vi "Main.vi"() -> ()   [LabVIEW 2013]
doc: "该连续测量范例项目在队列消息处理器模板的基础上实现。\n\n事件处理循环负责按用户界面操作生成对应的消息。\n\n消息处理循环负责对事件处理循环或其他消息生成的消息进行处理。其中还包括用于采集和记录消息处理循环的子VI，以及用于更新图表的循环。"
uses:
  Settings/Settings.ctl
  Acquisition/Hardware Configuration.ctl
  Acquisition/Signal Type.ctl
  Logging/Logging Configuration.ctl
  controls/UI Data.ctl
  controls/UI State.ctl
  support/Message Queue/Enqueue Message (Single).vi
  support/Message Queue/Enqueue Message (Array).vi
  <vilib>/Utility/error.llb/Error Cluster From Error Code.vi
  <vilib>/ErrorRing/Error Ring.xnode
  Acquisition/Acquisition.lvlib
  Logging/Logging.lvlib
  Settings/Settings.lvlib
  support/User Event - Stop/User Event - Stop.lvlib
  support/Message Queue/Message Queue.lvlib
panel:
  out "数据":waveform(dbl)[](graph)
  in  "设置":bool
  in  "开始":bool
  in  "停止":bool
  out "状态":string
  in  "退出":bool
  # "连续测量数据记录器"
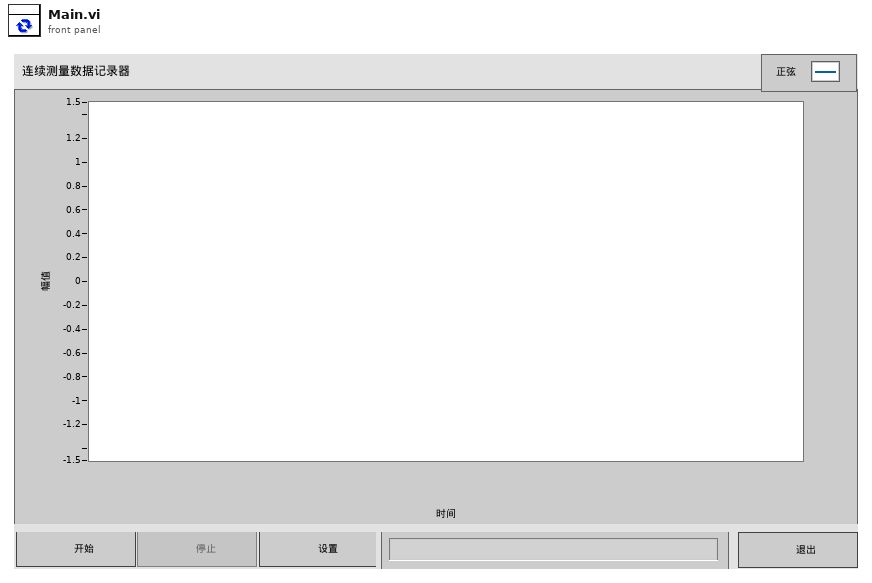
[diagram p1: front panel]
types:
  T1 = typedef "UI State.ctl" = enum16{"Idle", "Acquiring and Logging", "Waiting for Exit", "Waiting for Exit (Acq Stopped)", "Waiting for Exit (Log Stopped)", "Waiting for Stop", "Waiting for Stop (Acq Stopped)", "Waiting for Stop (Log Stopped)"}
  T2 = typedef "UI Data.ctl" = cluster{"开始引用":refnum<vi>, "停止引用":refnum<vi>, "设置引用":refnum<vi>, "退出引用":refnum<vi>, "状态引用":refnum<vi>, "数据引用":refnum<vi>}
  T3 = typedef "Settings.lvlib/Settings.ctl" = cluster{"硬件配置":T4, "记录配置":T6}
  T4 = typedef "Acquisition.lvlib/Hardware Configuration.ctl" = cluster{"硬件引用句柄<替换此项>":string, "信号类型<替换该项>":T5}
  T5 = typedef "Acquisition.lvlib/Signal Type.ctl" = enum16{"Sine Wave", "Square with Noise"}
  T6 = typedef "Logging.lvlib/Logging Configuration.ctl" = cluster{"记录文件基路径":path, "TDMS文件引用":refnum<k34>}
  T7 = typedef "Message Queue.lvlib/All Message Queues.ctl" = cluster{"UI":refnum<queue>, "采集":refnum<queue>, "记录":refnum<queue>}
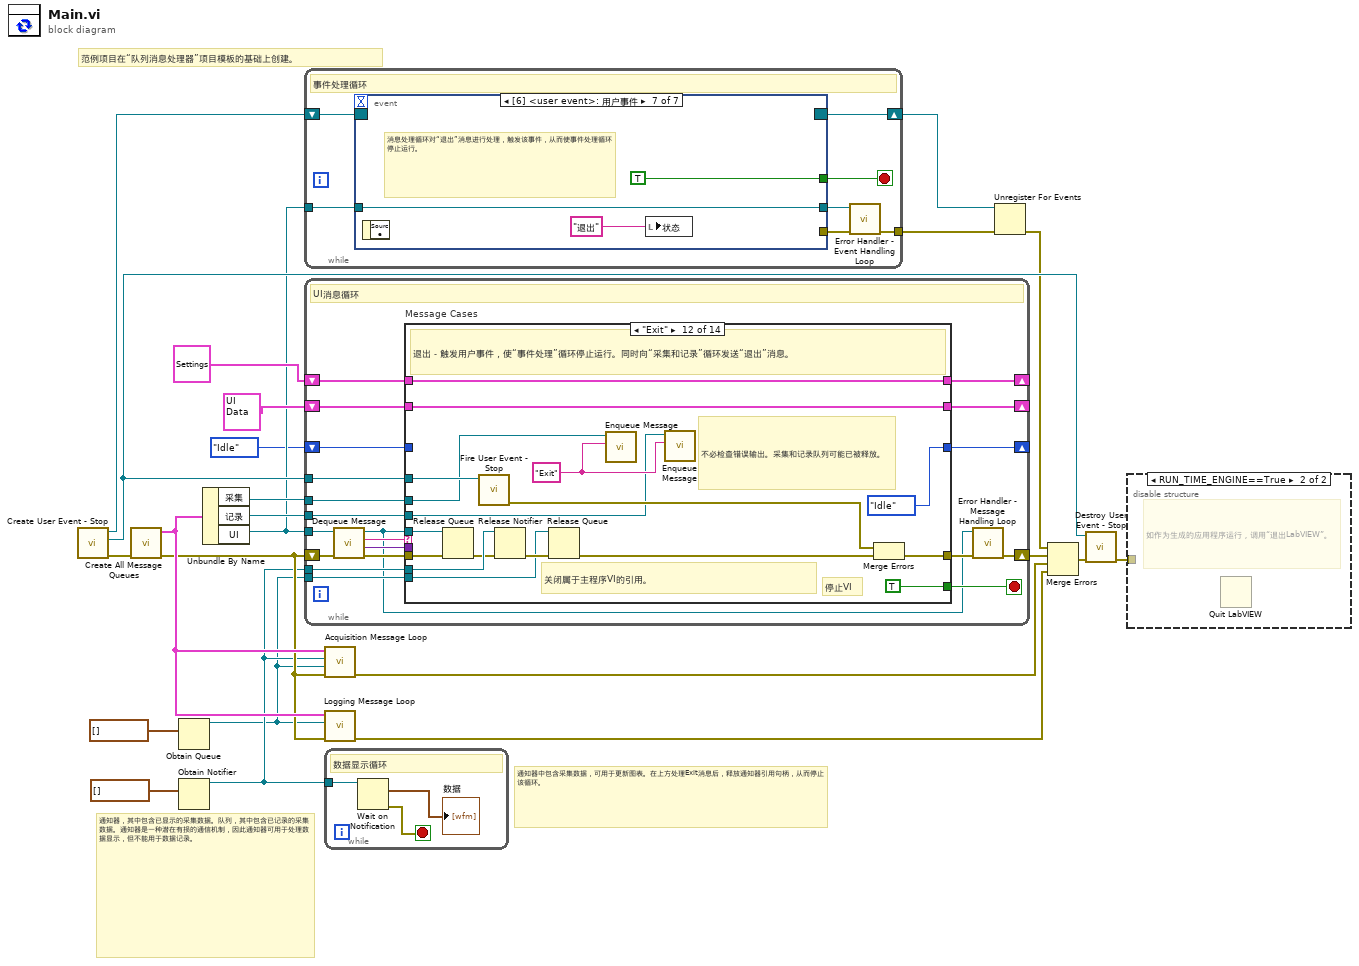
[diagram p0: block diagram]
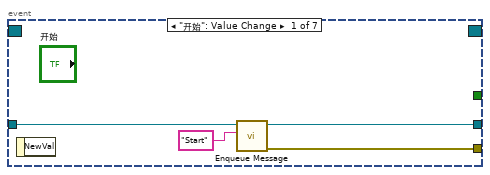
[diagram p3: hidden frame]
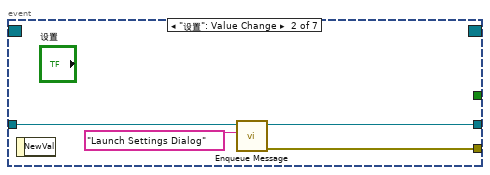
[diagram p4: hidden frame]
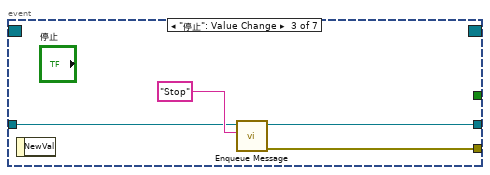
[diagram p5: hidden frame]
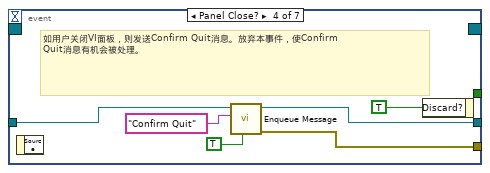
[diagram p6: hidden frame]
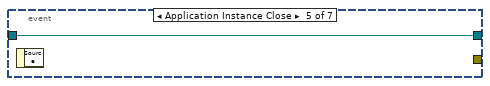
[diagram p7: hidden frame]
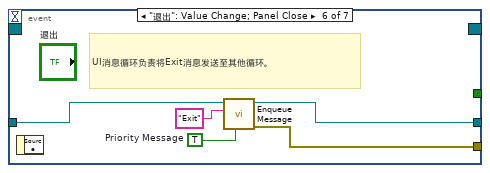
[diagram p8: hidden frame]
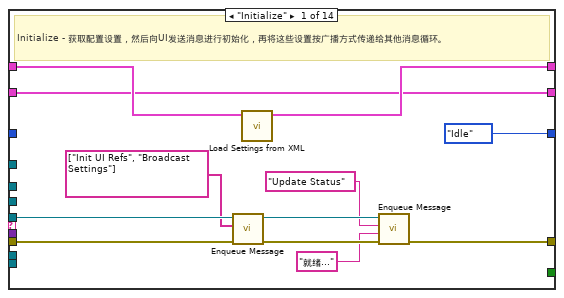
[diagram p9: hidden frame]
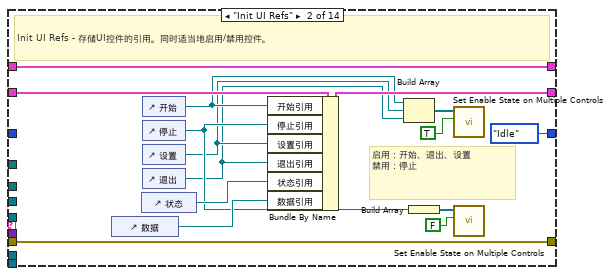
[diagram p10: hidden frame]
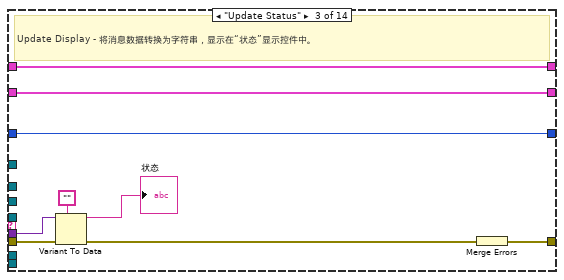
[diagram p11: hidden frame]
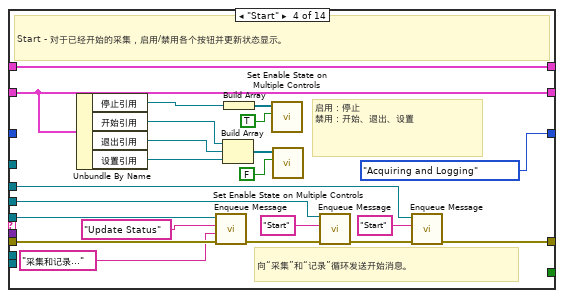
[diagram p12: hidden frame]
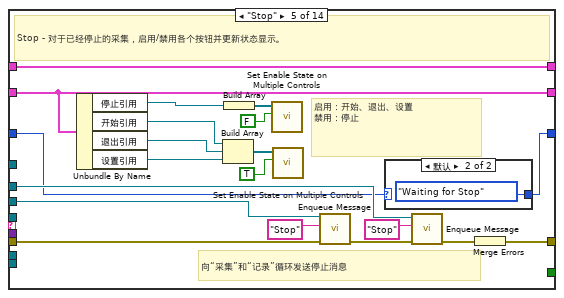
[diagram p13: hidden frame]
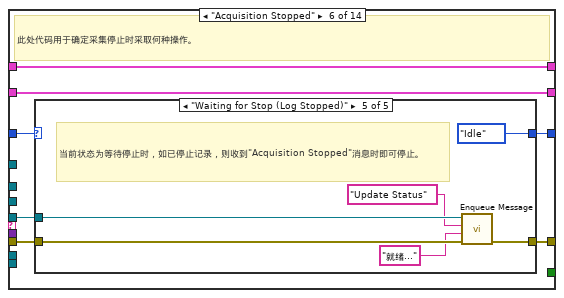
[diagram p15: hidden frame]
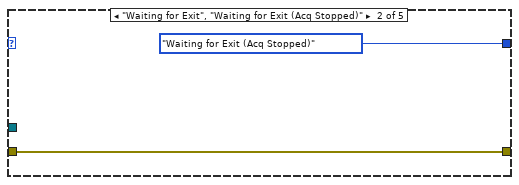
[diagram p17: hidden frame]
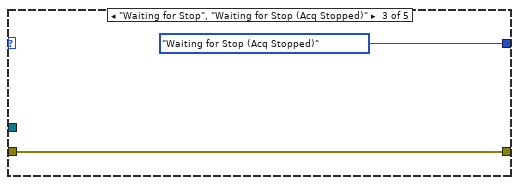
[diagram p18: hidden frame]
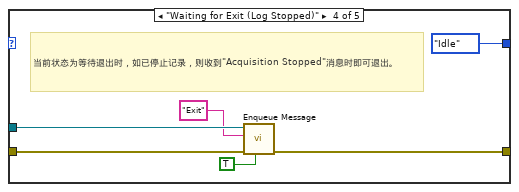
[diagram p19: hidden frame]
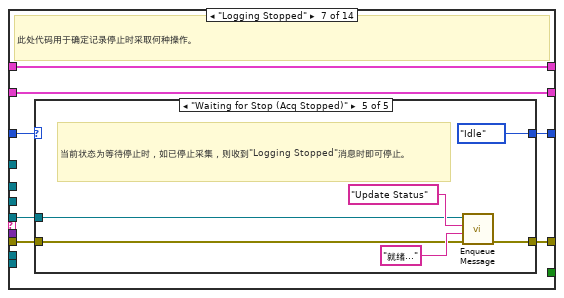
[diagram p20: hidden frame]
diagram:
  # "范例项目在“队列消息处理器”项目模板的基础上创建。"
  # "通知器，其中包含已显示的采集数据。队列，其中包含已记录的采集数据。通知器是一种潜在有损的通信机制，因此通知器可用于处理数据显示，但不能用于数据记录。"
  # "通知器中包含采集数据，可用于更新图表。在上方处理Exit消息后，释放通知器引用句柄，从而停止该循环。"
  n1 = call "Create User Event - Stop.vi"() -> ("error out"=w18:cluster{"状态":bool, "代码":i32, "源":string}, "用户事件－停止"=w20:refnum<user-event>, "停止事件注册引用句柄"=w21:refnum<event-registration>)  [unwired: 9 in]
  n2 = call "Create All Message Queues.vi"("error in (no error)"=w18) -> ("error out"=w15:cluster{"状态":bool, "代码":i32, "源":string}, "消息队列输出"=w17:T7)  [unwired: 9 in]
  n3 = Obtain Queue(element data type=waveform(dbl)[] []) -> (queue out=w4:refnum<queue>)  [unwired: 4 in, 2 out]
  n4 = Obtain Notifier(notification data type=waveform(dbl)[] []) -> (notifier out=w6:refnum<notifier>)  [unwired: 3 in, 2 out]
  n5 = Unbundle By Name(w17) -> ("采集"=w10:refnum<queue>, "记录"=w9:refnum<queue>, "UI"=w8:refnum<queue>)
  n6 = while {
    tunnel: w8 -> [w29]
    tunnel: [w26] -> w22
    shift-right: [w28] -> w12
    shift-left: w21 -> [w30]
    stop <- w27 stop-if-true
    # "事件处理循环"
    n7 = event shown="[6] <user event>: 用户事件" {
      selector: w30 -> [_ _ _ _ _ _ _]
      dyn-events: [_ _ _ _ _ _ _] -> w28
      timeout: _ -> [_ _ _ _ _ _ _]
      tunnel: [_ _ _ _ _ _ TRUE ("Discard?")] -> w27
      tunnel: w29 -> [w34 w36 w41 w46 w49 w51 w55]
      tunnel: [w32 w38 w40 w44 _ w54 _] -> w25
      tunnel: [w31 w35 w39 w45 w49 w50 w55] -> w24
      event "开始": Value Change {
        n8 = event-data() -> ()  [unwired: 1 in, 1 out]
        n9 = call-poly "Enqueue Message.vi"("消息"="Start" ("Message"), "消息队列"=w34) -> ("error out"=w32:cluster{"状态":bool, "代码":i32, "源":string}, "消息队列副本"=w31:refnum<queue>)  [unwired: 8 in]
      }
      event "设置": Value Change {
        n10 = event-data() -> ()  [unwired: 1 in, 1 out]
        n11 = call-poly "Enqueue Message.vi"("消息"="Launch Settings Dialog" ("Message"), "消息队列"=w36) -> ("error out"=w38:cluster{"状态":bool, "代码":i32, "源":string}, "消息队列副本"=w35:refnum<queue>)  [unwired: 8 in]
      }
      event "停止": Value Change {
        n12 = event-data() -> ()  [unwired: 1 in, 1 out]
        n13 = call-poly "Enqueue Message.vi"("消息"="Stop" ("Message"), "消息队列"=w41) -> ("error out"=w40:cluster{"状态":bool, "代码":i32, "源":string}, "消息队列副本"=w39:refnum<queue>)  [unwired: 8 in]
      }
      event Panel Close? {
        # "如用户关闭VI面板，则发送Confirm Quit消息。放弃本事件，使Confirm Quit消息有机会被处理。"
        n14 = event-data() -> ()  [unwired: 1 in, 1 out]
        n15 = call-poly "Enqueue Message.vi"("优先消息？(F)"=TRUE ("Priority Message? (F)"), "消息"="Confirm Quit" ("Message"), "消息队列"=w46) -> ("error out"=w44:cluster{"状态":bool, "代码":i32, "源":string}, "消息队列副本"=w45:refnum<queue>)  [unwired: 7 in]
        n16 = event-data("Discard?"=TRUE) -> ()  [unwired: 1 in, 1 out]
      }
      event Application Instance Close {
        n17 = event-data() -> ()  [unwired: 1 in, 1 out]
      }
      event "退出": Value Change; Panel Close {
        w52 = TRUE  # Priority Message
        # "UI消息循环负责将Exit消息发送至其他循环。"
        n18 = event-data() -> ()  [unwired: 1 in, 1 out]
        n19 = call-poly "Enqueue Message.vi"("优先消息？(F)"=w52, "消息"="Exit" ("Message"), "消息队列"=w51) -> ("error out"=w54:cluster{"状态":bool, "代码":i32, "源":string}, "消息队列副本"=w50:refnum<queue>)  [unwired: 7 in]
      }
      event User Event {
        # "消息处理循环对“退出”消息进行处理，触发该事件，从而使事件处理循环停止运行。"
        n20 = event-data() -> ()  [unwired: 1 in, 1 out]
        n21 = local write "状态"("退出" ("Exit String")) -> ()
      }
    }
    n22 = call "Error Handler - Event Handling Loop.vi"("error in (no error)"=w25, "消息队列"=w24) -> ("错误输入副本"=w26:cluster{"状态":bool, "代码":i32, "源":string})  [unwired: 8 in, 1 out]
  }
  n23 = while {
    tunnel: w8 -> [w71]
    tunnel: w20 -> [w76]
    shift-right: [w62] -> w23
    shift-left: w15 -> [w75]
    shift-right: [w70] -> _
    shift-left: T3 {"硬件配置"={"硬件引用句柄<替换此项>"="", "信号类型<替换该项>"=enum."Sine Wave"}, "记录配置"={"记录文件基路径"=path "", "TDMS文件引用"=refnum}} ("Settings") -> [w69]
    shift-right: [w67] -> _
    shift-left: T2 {"开始引用"=refnum, "停止引用"=refnum, "设置引用"=refnum, "退出引用"=refnum, "状态引用"=refnum, "数据引用"=refnum} ("Measurement UI Controls") -> [w68]
    tunnel: w10 -> [w66]
    tunnel: w9 -> [w65]
    tunnel: w6 -> [w64]
    tunnel: w4 -> [w63]
    shift-right: [w58] -> _
    shift-left: UI_State."Idle" ("UI State") -> [w59]
    stop <- w77 stop-if-true
    # "UI消息循环"
    n24 = call "Dequeue Message.vi"("error in (no error)"=w75, "消息队列"=w71) -> ("error out"=w74:cluster{"状态":bool, "代码":i32, "源":string}, "消息数据"=w72:variant, "消息"=w73:string, "消息队列副本"=w60:refnum<queue>)  [unwired: 6 in]
    n25 = case "Message Cases" shown="\"Exit\"" w73 {
      selector: w73 -> [_ _ _ _ _ _ _ _ _ _ _ _ _ w298]
      tunnel: w60 -> [w81 _ _ w135 _ w160 w185 _ w225 w239 w250 w281 _ _]
      tunnel: w74 -> [w80 w104 w112 w134 w154 w161 w186 w213 w227 w242 w249 w289 w296 _]
      tunnel: [w85 w104 w113 w117 w155 w158 w183 w219 w222 w238 w248 w290 w295 w297] -> w61
      tunnel: [_ _ _ _ _ _ _ _ _ _ _ TRUE _ _] -> w77
      tunnel: w72 -> [_ _ w111 _ _ _ _ _ _ w240 _ _ _ _]
      tunnel: w76 -> [_ _ _ _ _ _ _ _ _ _ _ w288 _ _]
      tunnel: [w88 w103 w107 w133 w153 w164 w189 w217 w224 w246 w253 w286 w294 w301] -> w70
      tunnel: w69 -> [w89 w103 w107 w133 w153 w164 w189 w217 w228 w246 w253 w286 w294 w301]
      tunnel: w68 -> [w82 w102 w106 w130 w152 w163 w188 w211 w221 w245 w252 w284 w293 w300]
      tunnel: [w82 w99 w106 w130 w152 w163 w188 w211 w221 w245 w252 w284 w293 w300] -> w67
      tunnel: w66 -> [_ _ _ w116 w139 _ _ w210 _ _ _ w283 _ _]
      tunnel: w65 -> [_ _ _ w119 w142 _ _ w209 _ _ _ w282 _ _]
      tunnel: w64 -> [_ _ _ _ _ _ _ _ _ _ _ w280 _ _]
      tunnel: w63 -> [_ _ _ _ _ _ _ _ _ _ _ w276 _ _]
      tunnel: w59 -> [_ _ w105 _ w136 w162 w187 w208 w220 w234 w251 _ w292 w299]
      tunnel: [UI_State."Idle" ("UI State") UI_State."Idle" ("UI State") w105 UI_State."Acquiring and Logging" ("UI State") w137 w159 w184 w208 w220 w234 w247 UI_State."Idle" ("UI State") w292 w299] -> w58
      frame "Initialize" {
        # "Initialize - 获取配置设置，然后向UI发送消息进行初始化，再将这些设置按广播方式传递给其他消息循环。"
        n26 = call-poly "Enqueue Message.vi"("error in (no error)"=w80, "消息数组"=string[] ["Init UI Refs", "Broadcast Settings"], "消息队列"=w81) -> ("error out"=w87:cluster{"状态":bool, "代码":i32, "源":string}, "消息队列副本"=w86:refnum<queue>)  [unwired: 7 in]
        n27 = call "Load Settings from XML.vi"("设置输入"=w89) -> ("设置输出"=w88:T3)  [unwired: 9 in, 1 out]
        n28 = call-poly "Enqueue Message.vi"("error in (no error)"=w87, "消息数据"="就绪..." ("Ready..."), "消息"="Update Status" ("Message"), "消息队列"=w86) -> ("error out"=w85:cluster{"状态":bool, "代码":i32, "源":string})  [unwired: 6 in, 1 out]
      }
      frame "Init UI Refs" {
        # "启用：开始、退出、设置\n禁用：停止"
        # "Init UI Refs - 存储UI控件的引用。同时适当地启用/禁用控件。"
        n29 = control-ref of="数据"() -> (w100:refnum<vi>)
        n30 = control-ref of="状态"() -> (w101:refnum<vi>)
        n31 = control-ref of="开始"() -> (w93:refnum<vi>)
        n32 = control-ref of="停止"() -> (w94:refnum<vi>)
        n33 = control-ref of="设置"() -> (w92:refnum<vi>)
        n34 = control-ref of="退出"() -> (w91:refnum<vi>)
        n35 = Bundle By Name(cluster=w102, "开始引用"=w93, "停止引用"=w94, "设置引用"=w92, "退出引用"=w91, "状态引用"=w101, "数据引用"=w100) -> (w99:T2)
        n36 = Build Array(w93, w92, w91) -> (w97:refnum<vi>[])
        n37 = Build Array(w94) -> (w96:refnum<vi>[])
        n38 = call "Set Enable State on Multiple Controls.vi"("启用？"=TRUE ("Enable?"), "控件"=w97) -> ()  [unwired: 10 in]
        n39 = call "Set Enable State on Multiple Controls.vi"("启用？"=FALSE ("Enable?"), "控件"=w96) -> ()  [unwired: 10 in]
      }
      frame "Update Status" {
        # "Update Display - 将消息数据转换为字符串，显示在“状态”显示控件中。"
        n40 = Variant To Data(error in=w112, type="", Variant=w111) -> (data=→"状态":string, error out=w109:errorcluster)
        n41 = Merge Errors(w109) -> (w113:errorcluster)
      }
      frame "Start" {
        # "向“采集”和“记录”循环发送开始消息。"
        # "启用：停止\n禁用：开始、退出、设置"
        # "Start - 对于已经开始的采集，启用/禁用各个按钮并更新状态显示。"
        n42 = Unbundle By Name(w130) -> ("停止引用"=w125:refnum<vi>, "开始引用"=w124:refnum<vi>, "退出引用"=w123:refnum<vi>, "设置引用"=w122:refnum<vi>)
        n43 = call-poly "Enqueue Message.vi"("error in (no error)"=w134, "消息数据"="采集和记录..." ("Acquiring and Logging..."), "消息"="Update Status" ("Message"), "消息队列"=w135) -> ("error out"=w121:cluster{"状态":bool, "代码":i32, "源":string})  [unwired: 6 in, 1 out]
        n44 = Build Array(w124, w123, w122) -> (w128:refnum<vi>[])
        n45 = Build Array(w125) -> (w127:refnum<vi>[])
        n46 = call "Set Enable State on Multiple Controls.vi"("启用？"=TRUE ("Enable?"), "控件"=w127) -> ()  [unwired: 10 in]
        n47 = call "Set Enable State on Multiple Controls.vi"("启用？"=FALSE ("Enable?"), "控件"=w128) -> ()  [unwired: 10 in]
        n48 = call-poly "Enqueue Message.vi"("error in (no error)"=w121, "消息"="Start" ("Message"), "消息队列"=w119) -> ("error out"=w118:cluster{"状态":bool, "代码":i32, "源":string})  [unwired: 7 in, 1 out]
        n49 = call-poly "Enqueue Message.vi"("error in (no error)"=w118, "消息"="Start" ("Message"), "消息队列"=w116) -> ("error out"=w117:cluster{"状态":bool, "代码":i32, "源":string})  [unwired: 7 in, 1 out]
      }
      frame "Stop" {
        # "向“采集”和“记录”循环发送停止消息"
        # "启用：开始、退出、设置\n禁用：停止"
        # "Stop - 对于已经停止的采集，启用/禁用各个按钮并更新状态显示。"
        n50 = Unbundle By Name(w152) -> ("停止引用"=w147:refnum<vi>, "开始引用"=w146:refnum<vi>, "退出引用"=w145:refnum<vi>, "设置引用"=w144:refnum<vi>)
        n51 = Build Array(w146, w145, w144) -> (w150:refnum<vi>[])
        n52 = Build Array(w147) -> (w149:refnum<vi>[])
        n53 = call "Set Enable State on Multiple Controls.vi"("启用？"=FALSE ("Enable?"), "控件"=w149) -> ()  [unwired: 10 in]
        n54 = call "Set Enable State on Multiple Controls.vi"("启用？"=TRUE ("Enable?"), "控件"=w150) -> ()  [unwired: 10 in]
        n55 = call-poly "Enqueue Message.vi"("error in (no error)"=w154, "消息"="Stop" ("Message"), "消息队列"=w142) -> ("error out"=w141:cluster{"状态":bool, "代码":i32, "源":string})  [unwired: 7 in, 1 out]
        n56 = case shown="默认" w136 {
          selector: w136 -> [w156 _]
          tunnel: [w156 UI_State."Waiting for Stop" ("UI State")] -> w137
          frame "Waiting for Exit" {
          }
          frame Default {
          }
        }
        n57 = call-poly "Enqueue Message.vi"("error in (no error)"=w141, "消息"="Stop" ("Message"), "消息队列"=w139) -> ("error out"=w140:cluster{"状态":bool, "代码":i32, "源":string})  [unwired: 7 in, 1 out]
        n58 = Merge Errors(w140) -> (w155:errorcluster)
      }
      frame "Acquisition Stopped" {
        # "此处代码用于确定采集停止时采取何种操作。"
        n59 = case shown="\"Waiting for Stop (Log Stopped)\"" w162 {
          selector: w162 -> [w166 _ _ _ _]
          tunnel: w161 -> [w165 w168 w170 w176 w182]
          tunnel: w160 -> [_ _ _ w174 w179]
          tunnel: [w166 UI_State."Waiting for Exit (Acq Stopped)" ("UI State") UI_State."Waiting for Stop (Acq Stopped)" ("UI State") UI_State."Idle" ("UI State") UI_State."Idle" ("UI State")] -> w159
          tunnel: [w165 w168 w170 w175 w180] -> w158
          frame Default {
          }
          frame "Waiting for Exit", "Waiting for Exit (Acq Stopped)" {
          }
          frame "Waiting for Stop", "Waiting for Stop (Acq Stopped)" {
          }
          frame "Waiting for Exit (Log Stopped)" {
            # "当前状态为等待退出时，如已停止记录，则收到\"Acquisition Stopped\"消息时即可退出。"
            n60 = call-poly "Enqueue Message.vi"("优先消息？(F)"=TRUE ("Priority Message? (F)"), "error in (no error)"=w176, "消息"="Exit", "消息队列"=w174) -> ("error out"=w175:cluster{"状态":bool, "代码":i32, "源":string})  [unwired: 6 in, 1 out]
          }
          frame "Waiting for Stop (Log Stopped)" {
            # "当前状态为等待停止时，如已停止记录，则收到\"Acquisition Stopped\"消息时即可停止。"
            n61 = call-poly "Enqueue Message.vi"("error in (no error)"=w182, "消息数据"="就绪..." ("Ready..."), "消息"="Update Status" ("Message"), "消息队列"=w179) -> ("error out"=w180:cluster{"状态":bool, "代码":i32, "源":string})  [unwired: 6 in, 1 out]
          }
        }
      }
      frame "Logging Stopped" {
        # "此处代码用于确定记录停止时采取何种操作。"
        n62 = case shown="\"Waiting for Stop (Acq Stopped)\"" w187 {
          selector: w187 -> [w191 _ _ _ _]
          tunnel: w186 -> [w190 w193 w195 w201 w204]
          tunnel: w185 -> [_ _ _ w199 w203]
          tunnel: [w191 UI_State."Waiting for Exit (Log Stopped)" ("UI State") UI_State."Waiting for Stop (Log Stopped)" ("UI State") UI_State."Idle" ("UI State") UI_State."Idle" ("UI State")] -> w184
          tunnel: [w190 w193 w195 w200 w202] -> w183
          frame Default {
          }
          frame "Waiting for Exit", "Waiting for Exit (Log Stopped)" {
          }
          frame "Waiting for Stop", "Waiting for Stop (Log Stopped)" {
          }
          frame "Waiting for Exit (Acq Stopped)" {
            # "当前状态为等待退出时，如已停止采集，则收到\"Logging Stopped\"消息时即可退出。"
            n63 = call-poly "Enqueue Message.vi"("优先消息？(F)"=TRUE ("Priority Message? (F)"), "error in (no error)"=w201, "消息"="Exit", "消息队列"=w199) -> ("error out"=w200:cluster{"状态":bool, "代码":i32, "源":string})  [unwired: 6 in, 1 out]
          }
          frame "Waiting for Stop (Acq Stopped)" {
            # "当前状态为等待停止时，如已停止采集，则收到\"Logging Stopped\"消息时即可停止。"
            n64 = call-poly "Enqueue Message.vi"("error in (no error)"=w204, "消息数据"="就绪..." ("Ready..."), "消息"="Update Status" ("Message"), "消息队列"=w203) -> ("error out"=w202:cluster{"状态":bool, "代码":i32, "源":string})  [unwired: 6 in, 1 out]
          }
        }
      }
      frame "Broadcast settings" {
        w212 = "Update Settings" ("Message")
        # "Broadcast settings - 向“记录和采集”消息队列发送“更新设置”消息。"
        n65 = Unbundle By Name(w217) -> ("硬件配置"=w216:T4, "记录配置"=w215:T6)
        n66 = call-poly "Enqueue Message.vi"("消息数据"=w216, "消息"=w212, "消息队列"=w210) -> ("error out"=w218:cluster{"状态":bool, "代码":i32, "源":string})  [unwired: 7 in, 1 out]
        n67 = call-poly "Enqueue Message.vi"("error in (no error)"=w218, "消息数据"=w215, "消息"=w212, "消息队列"=w209) -> ("error out"=w214:cluster{"状态":bool, "代码":i32, "源":string})  [unwired: 6 in, 1 out]
        n68 = Merge Errors(w214, w213) -> (w219:errorcluster)
      }
      frame "Launch Settings Dialog" {
        # "Launch Settings Dialog - 用户单击“设置”按钮时，启动设置对话框。"
        n69 = call "Settings Dialog.vi"("error in (no error)"=w227, "设置输入"=w228) -> ("error out"=w223:cluster{"状态":bool, "代码":i32, "源":string}, "取消？"=w226:bool, "设置输出"=w224:T3)  [unwired: 6 in, 1 out]
        n70 = case shown="假" w226 {
          tunnel: w225 -> [w232 _]
          tunnel: w223 -> [w231 w233]
          tunnel: [w230 w233] -> w222
          frame False {
            n71 = call-poly "Enqueue Message.vi"("error in (no error)"=w231, "消息"="Broadcast Settings" ("Message"), "消息队列"=w232) -> ("error out"=w230:cluster{"状态":bool, "代码":i32, "源":string})  [unwired: 7 in, 1 out]
          }
          frame True {
          }
        }
      }
      frame "Error" {
        # "Error - 检查错误消息数据及其响应。本应用程序中，该消息由每个循环结束处的“错误处理”VI发送。"
        n72 = Variant To Data(error in=w242, type=errorcluster {"status"=FALSE, "code"=0, "source"=""} ("error constant"), Variant=w240) -> (data=w244:errorcluster, error out=w241:errorcluster)
        n73 = call <vilib>:"Simple Error Handler.vi"("error in (no error)"=w244) -> ()  [unwired: 4 in, 5 out]
        n74 = call-poly "Enqueue Message.vi"("优先消息？(F)"=TRUE ("Priority Message? (F)"), "消息"="Exit", "消息队列"=w239) -> ("error out"=w237:cluster{"状态":bool, "代码":i32, "源":string})  [unwired: 7 in, 1 out]
        n75 = Merge Errors(w237, w241) -> (w238:errorcluster)
      }
      frame "Confirm Quit" {
        # "Confirm Quit - 该消息用于确认用户是否需要退出应用程序。"
        n76 = case shown="\"Acquiring and Logging\"" w251 {
          tunnel: w250 -> [w259 w263]
          tunnel: w249 -> [w258 w262]
          tunnel: [w257 w261] -> w248
          tunnel: [UI_State."Idle" ("UI State") w260] -> w247
          frame Default {
            # "如收到'Confirm Quit'消息时系统处于空闲状态，则不需要弹出确认提示。"
            n77 = call-poly "Enqueue Message.vi"("优先消息？(F)"=TRUE ("Priority Message? (F)"), "error in (no error)"=w258, "消息"="Exit", "消息队列"=w259) -> ("error out"=w257:cluster{"状态":bool, "代码":i32, "源":string})  [unwired: 6 in, 1 out]
          }
          frame "Acquiring and Logging" {
            n78 = Two Button Dialog(message="采集仍在执行中，是否确定退出？" ("Confirm Quit Message"), 1:"否" ("No"), 2:"是" ("Yes")) -> (T button?=w264:bool)
            n79 = case shown="真" w264 {
              tunnel: w263 -> [_ w273]
              tunnel: w262 -> [w269 w274]
              tunnel: [w269 w272] -> w261
              tunnel: [UI_State."Acquiring and Logging" ("UI State") UI_State."Waiting for Exit" ("UI State")] -> w260
              frame False {
                # "用户不希望退出。"
              }
              frame True {
                n80 = call-poly "Enqueue Message.vi"("error in (no error)"=w274, "消息"="Stop", "消息队列"=w273) -> ("error out"=w272:cluster{"状态":bool, "代码":i32, "源":string})  [unwired: 7 in, 1 out]
              }
            }
          }
        }
      }
      frame "Exit" {
        w285 = "Exit" ("Message")
        # "不必检查错误输出。采集和记录队列可能已被释放。"
        # "关闭属于主程序VI的引用。"
        # "停止VI"
        # "退出－触发用户事件，使“事件处理”循环停止运行。同时向“采集和记录”循环发送“退出”消息。"
        n81 = Release Queue(queue=w281, error in (no error)=w289) -> (error out=w279:errorcluster)  [unwired: 1 in, 2 out]
        n82 = call "Fire User Event - Stop.vi"("用户事件－停止"=w288) -> ("error out"=w287:cluster{"状态":bool, "代码":i32, "源":string})  [unwired: 10 in]
        n83 = Release Notifier(notifier=w280, error in (no error)=w279) -> (error out=w278:errorcluster)  [unwired: 1 in, 2 out]
        n84 = Release Queue(queue=w276, error in (no error)=w278) -> (error out=w277:errorcluster)  [unwired: 1 in, 2 out]
        n85 = call-poly "Enqueue Message.vi"("消息"=w285, "消息队列"=w283) -> ()  [unwired: 8 in, 2 out]
        n86 = call-poly "Enqueue Message.vi"("消息"=w285, "消息队列"=w282) -> ()  [unwired: 8 in, 2 out]
        n87 = Merge Errors(w287, w277) -> (w290:errorcluster)
      }
      frame "---Copy This Frame---" {
        # "如需创建新消息，可创建该帧的副本。在副本中，将本注释更改为对应消息的注释。"
        n88 = Merge Errors(w296) -> (w295:errorcluster)
      }
      frame Default {
        # "如得到的消息未经任何分支定义，则运行“默认”分支。输出程序错误。"
        n89 = xnode "Error Ring"("参数 0"=w298) -> ("错误输出"=w297:errorcluster)
      }
    }
    n90 = call "Error Handler - Message Handling Loop.vi"("error in (no error)"=w61, "消息队列"=w60) -> ("错误输入副本"=w62:cluster{"状态":bool, "代码":i32, "源":string})  [unwired: 8 in, 1 out]
  }
  n91 = call "Acquisition Message Loop.vi"("error in (no error)"=w15, "数据队列"=w4, "数据通知器"=w6, "消息队列"=w17) -> ("error out"=w19:cluster{"状态":bool, "代码":i32, "源":string})  [unwired: 7 in]
  n92 = call "Logging Message Loop.vi"("error in (no error)"=w15, "数据队列"=w4, "消息队列"=w17) -> ("error out"=w16:cluster{"状态":bool, "代码":i32, "源":string})  [unwired: 8 in]
  n93 = while "Data Display Loop" {
    tunnel: w6 -> [w311]
    stop <- w309 stop-if-true
    # "数据显示循环"
    n94 = Wait on Notification(notifier=w311) -> (notification=→"数据":waveform(dbl)[], error out=w309:errorcluster)  [unwired: 3 in, 2 out]
  }
  n95 = Unregister For Events(event registration refnum=w12, error in=w22) -> (error out=w13:errorcluster)
  n96 = Merge Errors(w13, w23, w19, w16) -> (w1:errorcluster)
  n97 = call "Destroy User Event - Stop.vi"("error in (no error)"=w1, "用户事件－停止"=w20) -> ("error out"=w3:cluster{"状态":bool, "代码":i32, "源":string})  [unwired: 9 in]
  n98 = disable-structure shown="RUN_TIME_ENGINE==True" {
    disable-tunnel: w3 -> [_ _]
    frame condition #0 (active) {
    }
    frame condition #1 {
      # "如作为生成的应用程序运行，调用“退出LabVIEW”。"
      n99 = Quit LabVIEW() -> ()  [unwired: 1 in]
    }
  }
